vi "WriteMessage.vi"(0 "reference":refnum<class "VdTcpIP.lvclass">, 2 "Message":string, 3 "timeout ms (25000)":i32=25000, 4 "Binary(F)":bool, 5 "error in (no error)":errorcluster) -> (14 "reference out":refnum<class "VdTcpIP.lvclass">, 17 "Reconnected":bool, 19 "error out":errorcluster)   [LabVIEW 2020, in "VdTcpIP.lvclass"]
doc: "Write a simple message to a connection"
uses:
  VdTcpIP.lvclass
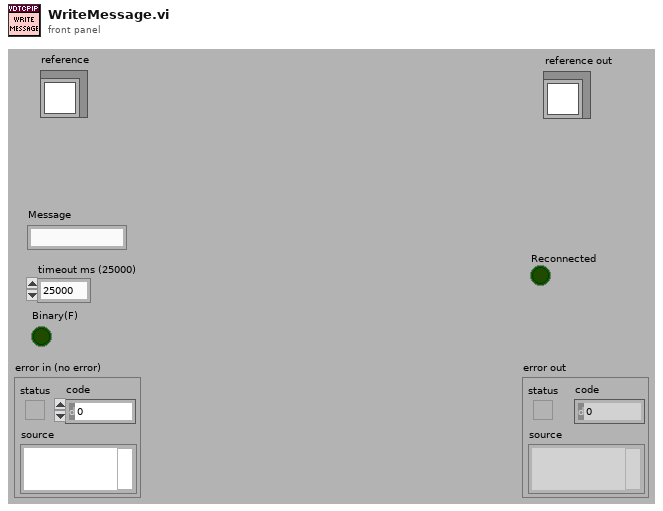
[diagram p1: front panel]
types:
  T1 = typedef "VdTcpIP.lvclass/ObjectAttributes.ctl" = cluster{"IP-Address":string, "Port":u16, "Connection":refnum<k5>, "Listener":refnum<k5>, "ListenerConnection":refnum<k5>, "Listner":bool, "ListnerProcessRunning":bool, "InConnections":refnum<k5>[], "InConnectionsIP":string[], "InConnectionAdded":refnum<notifier>, "RunVIOnNewConnection":variant, "DataToNewConnectionVI":cluster{"ControlName":string, "ControlValue":variant}[], "WebServicesURL_Location(http://...)":string, "WebServicesPostWebPage(*.asmx)":string, "Semaphore":T2, "AutoReConnectTimes":i32, "AutoReConnectInterval(ms)":i32, "ConnectionTimeout":i32}
  T2 = typedef "Semaphore RefNum" = refnum<k1>
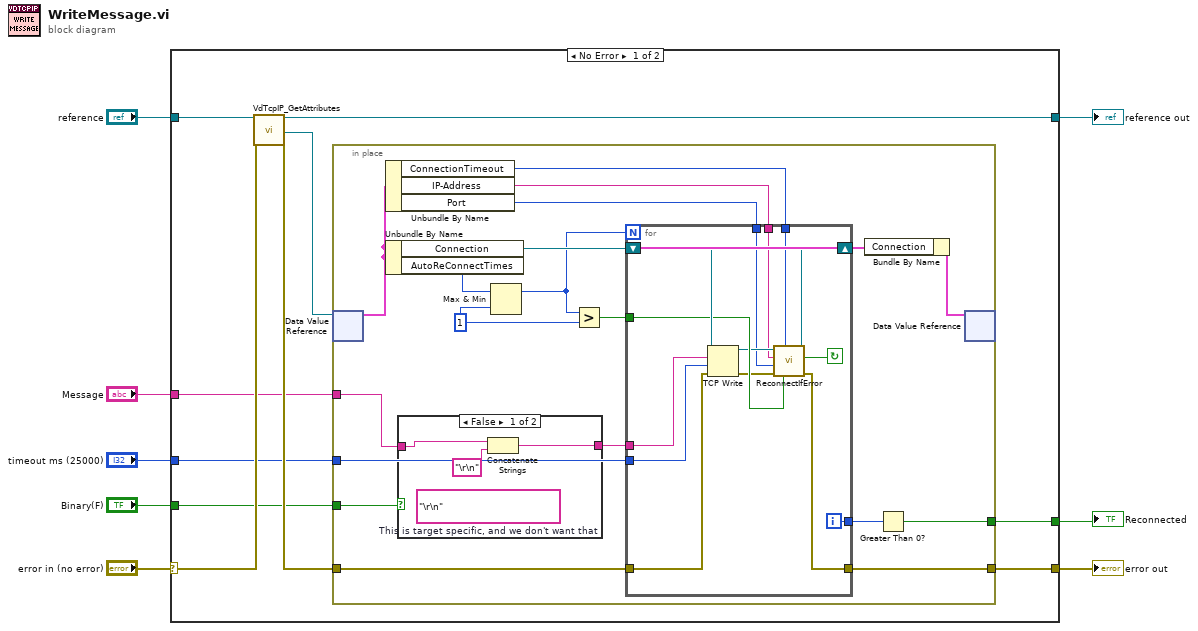
[diagram p0: block diagram]
diagram:
  n1 = case shown="No Error" "error in (no error)" {
    selector: "error in (no error)" -> [w18 w56]
    tunnel: "reference" -> [w11 w57]
    tunnel: [w9 w56] -> w6
    tunnel: [w10 w57] -> w5
    tunnel: "Message" -> [w16 _]
    tunnel: "timeout ms (25000)" -> [w15 _]
    tunnel: "Binary(F)" -> [w14 _]
    tunnel: [w12 _] -> w1
    frame No Error {
      n2 = call "VdTcpIP_GetAttributes.vi"("reference in"=w11, "error in (no error)"=w18) -> ("reference out"=w10:refnum<class "VdTcpIP.lvclass">, "DataRef"=w13:refnum<data-value>, "error out"=w17:errorcluster)  [unwired: 1 in, 14 out]
      n3 = in-place {
        in-place-border: w17 -> [w37]
        in-place-border: [w36] -> w9
        in-place-border: w16 -> [w20]
        in-place-border: w15 -> [w34]
        in-place-border: w14 -> [w21]
        in-place-border: [w22] -> w12
        w32 = 1 ("x")
        n4 = in-place-dvr #1(w13) -> (w26:T1)  [unwired: 1 out]
        n5 = Unbundle By Name(w26) -> ("ConnectionTimeout"=w29:i32, "IP-Address"=w28:string, "Port"=w27:u16)
        n6 = Unbundle By Name(w26) -> ("Connection"=w35:refnum<k5>, "AutoReConnectTimes"=w33:i32)
        n7 = case shown="False" w21 {
          tunnel: w20 -> [w40 w41]
          tunnel: [w39 w41] -> w19
          frame False {
            (unwired) "\r\n"  # This is target specific, and we don't want that
            n8 = Concatenate Strings(w40, "\r\n" ("string")) -> (w39:string)
          }
          frame True {
          }
        }
        n9 = Max & Min(x=w33, y=w32) -> (max(x,y)=w31:i32)  [unwired: 1 out]
        n10 = Greater?(x=w31, y=w32) -> (0:w30:bool)
        n11 = for {
          N: w31 -> [_]
          tunnel: w34 -> [w53]
          tunnel: w30 -> [w52]
          tunnel: w37 -> [w55]
          tunnel: [w50] -> w36
          tunnel: w29 -> [w48]
          shift-right: [w46] -> w24
          shift-left: w35 -> [w54]
          tunnel: w28 -> [w45]
          tunnel: w27 -> [w44]
          tunnel: [w43] -> w23
          tunnel: w19 -> [w42]
          i -> [w43]
          stop <- w49 continue-if-true
          n12 = TCP Write(connection ID=w54, data in=w42, error in (no error)=w55, 9:w53) -> (connection ID out=w47:refnum<k5>, error out=w51:errorcluster)  [unwired: 1 out]
          n13 = call "ReconnectIfError.vi"("TryReconnect"=w52, "ConnectionTimeout"=w48, "error in (no error)"=w51, "Port"=w44, "IP-Address"=w45, "TCP Network Connection in"=w47) -> ("error out"=w50:errorcluster, "TryAgain(Managed to Reconnect, and TryReconnect is True)"=w49:bool, "TCP Network Connection out"=w46:refnum<k5>)  [unwired: 3 in]
        }
        n14 = Bundle By Name(cluster=w26, "Connection"=w24) -> (w25:T1)
        n15 = Greater Than 0?(x=w23) -> (x > 0?=w22:bool)
        n16 = in-place-dvr #1(w25) -> ()  [unwired: 2 out]
      }
    }
    frame Error {
    }
  }
  "reference out" <- w5
  "error out" <- w6
  "Reconnected" <- w1
